vi "水样数据发送帧.vi"(10 "数据类别":u16(ring) items=["水样数据"=0, "标样数据"=1, "零点核查数据"=2, "跨度核查数据"=3, "环境变量"=4, "水样数据补传"=16, "标样核查数据补传"=17, "零点核查数据补传"=18, "跨度核查数据补传"=19], 11 "用户地址":string) -> (1 "非x？":bool, 2 "报文长度":i32, 3 "字符串":string)   [LabVIEW 2016, in "环境动力监测库.lvlib" / "NMEA.lvlib"]
uses:
  NMEA.lvlib
panel:
  out "data":T1 {"数组"."标识" items=["N"=1, "T"=2, "L"=3, "D"=4, "Z"=5, "M"=6, "hd"=7]; "数组"."污染物" items=["水温"=1, "浊度"=2, "DO"=3, "pH"=4, "ORP"=5, "比电导率"=6, "叶绿素a"=7, "氨氮"=8, "亚硝氮"=9, "硫化物"=10, "电压"=11, "温度"=12, "湿度"=13, "GPS经度"=14, "GPS纬度"=15, "BD经度"=16, "BD纬度"=17]; "数据类别" items=["水样数据"=0, "标样数据"=1, "零点核查数据"=2, "跨度核查数据"=3, "环境变量"=4, "水样数据补传"=16, "标样核查数据补传"=17, "零点核查数据补传"=18, "跨度核查数据补传"=19]}
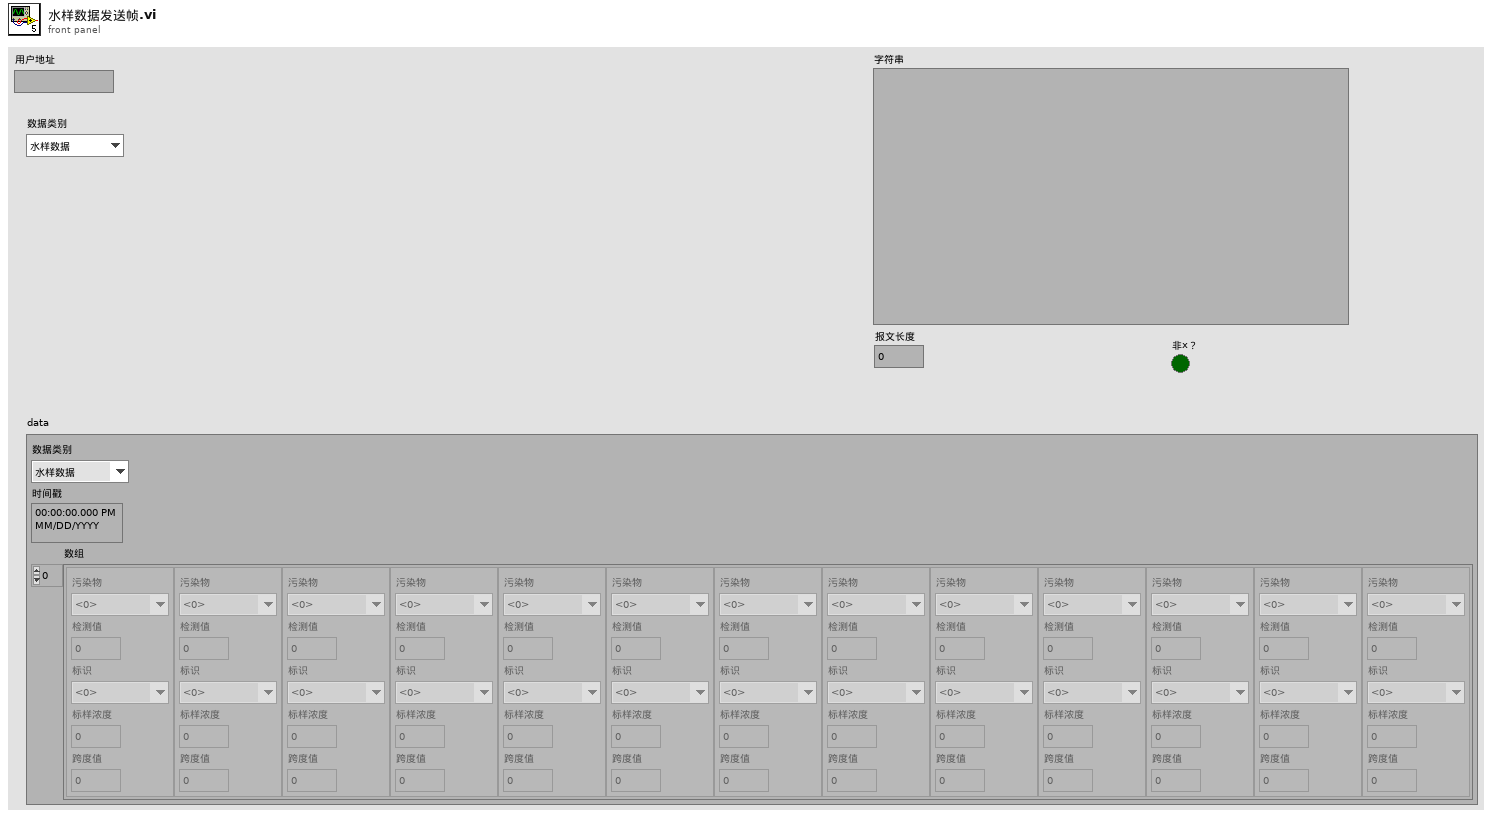
[diagram p1: front panel]
types:
  T1 = cluster{"数据类别":u16, "时间戳":timestamp, "数组":cluster{"污染物":u16, "检测值":dbl, "标识":u16, "标样浓度":dbl, "跨度值":dbl}[]}
  T2 = cluster{"污染物":u16, "检测值":dbl, "标识":u16, "标样浓度":dbl, "跨度值":dbl}[]
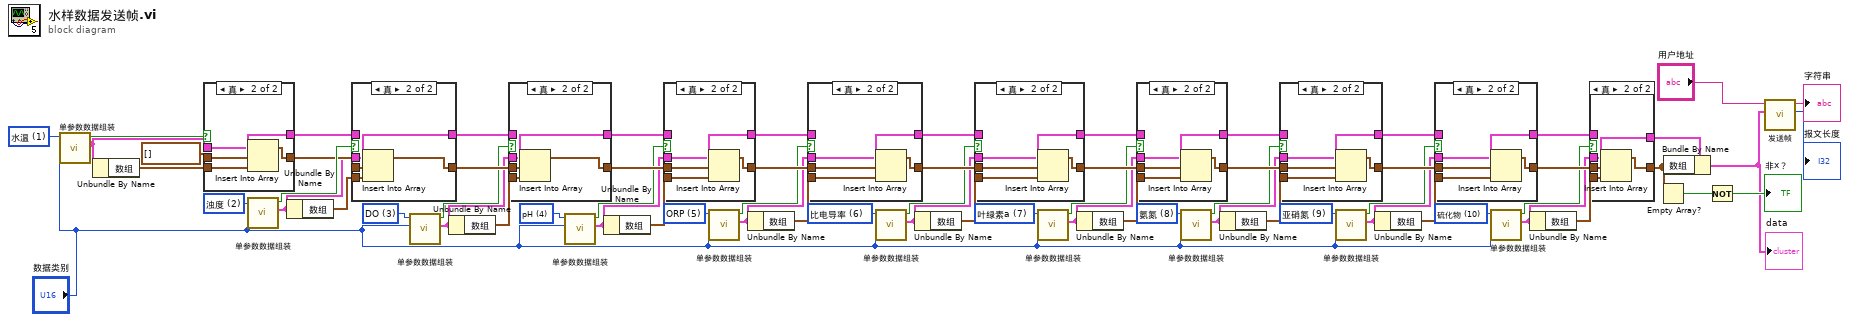
[diagram p0: block diagram]
diagram:
  w59 = u16 7 items=["水温"=1, "浊度"=2, "DO"=3, "pH"=4, "ORP"=5, "比电导率"=6, "叶绿素a"=7, "氨氮"=8, "亚硝氮"=9, "硫化物"=10, "经度"=11, "维度"=12, "电压"=13] ("污染物")
  w60 = u16 6 items=["水温"=1, "浊度"=2, "DO"=3, "pH"=4, "ORP"=5, "比电导率"=6, "叶绿素a"=7, "氨氮"=8, "亚硝氮"=9, "硫化物"=10, "经度"=11, "维度"=12, "电压"=13] ("污染物")
  w61 = u16 5 items=["水温"=1, "浊度"=2, "DO"=3, "pH"=4, "ORP"=5, "比电导率"=6, "叶绿素a"=7, "氨氮"=8, "亚硝氮"=9, "硫化物"=10, "经度"=11, "维度"=12, "电压"=13] ("污染物")
  w62 = u16 4 items=["水温"=1, "浊度"=2, "DO"=3, "pH"=4, "ORP"=5, "比电导率"=6, "叶绿素a"=7, "氨氮"=8, "亚硝氮"=9, "硫化物"=10, "经度"=11, "维度"=12, "电压"=13] ("污染物")
  w63 = u16 3 items=["水温"=1, "浊度"=2, "DO"=3, "pH"=4, "ORP"=5, "比电导率"=6, "叶绿素a"=7, "氨氮"=8, "亚硝氮"=9, "硫化物"=10, "经度"=11, "维度"=12, "电压"=13] ("污染物")
  w64 = u16 2 items=["水温"=1, "浊度"=2, "DO"=3, "pH"=4, "ORP"=5, "比电导率"=6, "叶绿素a"=7, "氨氮"=8, "亚硝氮"=9, "硫化物"=10, "经度"=11, "维度"=12, "电压"=13] ("污染物")
  w65 = u16 1 items=["水温"=1, "浊度"=2, "DO"=3, "pH"=4, "ORP"=5, "比电导率"=6, "叶绿素a"=7, "氨氮"=8, "亚硝氮"=9, "硫化物"=10, "经度"=11, "维度"=12, "电压"=13] ("污染物")
  w66 = u16 10 items=["水温"=1, "浊度"=2, "DO"=3, "pH"=4, "ORP"=5, "比电导率"=6, "叶绿素a"=7, "氨氮"=8, "亚硝氮"=9, "硫化物"=10, "经度"=11, "维度"=12, "电压"=13] ("污染物")
  w67 = u16 9 items=["水温"=1, "浊度"=2, "DO"=3, "pH"=4, "ORP"=5, "比电导率"=6, "叶绿素a"=7, "氨氮"=8, "亚硝氮"=9, "硫化物"=10, "经度"=11, "维度"=12, "电压"=13] ("污染物")
  w68 = u16 8 items=["水温"=1, "浊度"=2, "DO"=3, "pH"=4, "ORP"=5, "比电导率"=6, "叶绿素a"=7, "氨氮"=8, "亚硝氮"=9, "硫化物"=10, "经度"=11, "维度"=12, "电压"=13] ("污染物")
  n1 = call "单参数数据组装.vi"("数据类别"="数据类别", "污染物"=w65) -> ("data"=w28:T1, "布尔"=w58:bool)  [unwired: 8 in]
  n2 = Unbundle By Name(w28) -> ("数组"=w39:T2)
  n3 = case shown="真" w58 {
    tunnel: w39 -> [_ w74]
    tunnel: T2 [] ("数组") -> [w70 w73]
    tunnel: [w70 w72] -> w56
    tunnel: w28 -> [w69 w71]
    tunnel: [w69 w71] -> w27
    frame False {
    }
    frame True {
      n4 = Insert Into Array(array=w73, new element=w74) -> (w72:T2)  [unwired: 1 in]
    }
  }
  n5 = call "单参数数据组装.vi"("数据类别"="数据类别", "污染物"=w64) -> ("data"=w17:T1, "布尔"=w57:bool)  [unwired: 8 in]
  n6 = Unbundle By Name(w17) -> ("数组"=w38:T2)
  n7 = case shown="真" w57 {
    tunnel: w38 -> [_ w80]
    tunnel: w56 -> [w76 w79]
    tunnel: [w76 w78] -> w55
    tunnel: [w75 w77] -> w26
    tunnel: w27 -> [w75 _]
    tunnel: w17 -> [_ w77]
    frame False {
    }
    frame True {
      n8 = Insert Into Array(array=w79, new element=w80) -> (w78:T2)  [unwired: 1 in]
    }
  }
  n9 = call "单参数数据组装.vi"("数据类别"="数据类别", "污染物"=w63) -> ("data"=w16:T1, "布尔"=w50:bool)  [unwired: 8 in]
  n10 = Unbundle By Name(w16) -> ("数组"=w37:T2)
  n11 = case shown="真" w50 {
    tunnel: w37 -> [_ w86]
    tunnel: w55 -> [w82 w85]
    tunnel: [w82 w84] -> w54
    tunnel: w26 -> [w81 _]
    tunnel: [w81 w83] -> w25
    tunnel: w16 -> [_ w83]
    frame False {
    }
    frame True {
      n12 = Insert Into Array(array=w85, new element=w86) -> (w84:T2)  [unwired: 1 in]
    }
  }
  n13 = call "单参数数据组装.vi"("数据类别"="数据类别", "污染物"=w62) -> ("data"=w15:T1, "布尔"=w49:bool)  [unwired: 8 in]
  n14 = Unbundle By Name(w15) -> ("数组"=w36:T2)
  n15 = case shown="真" w49 {
    tunnel: w36 -> [_ w92]
    tunnel: w54 -> [w88 w91]
    tunnel: [w88 w90] -> w52
    tunnel: w25 -> [w87 _]
    tunnel: [w87 w89] -> w24
    tunnel: w15 -> [_ w89]
    frame False {
    }
    frame True {
      n16 = Insert Into Array(array=w91, new element=w92) -> (w90:T2)  [unwired: 1 in]
    }
  }
  n17 = call "单参数数据组装.vi"("数据类别"="数据类别", "污染物"=w61) -> ("data"=w14:T1, "布尔"=w48:bool)  [unwired: 8 in]
  n18 = Unbundle By Name(w14) -> ("数组"=w35:T2)
  n19 = case shown="真" w48 {
    tunnel: w35 -> [_ w98]
    tunnel: w52 -> [w94 w97]
    tunnel: [w94 w96] -> w53
    tunnel: w24 -> [w93 _]
    tunnel: [w93 w95] -> w23
    tunnel: w14 -> [_ w95]
    frame False {
    }
    frame True {
      n20 = Insert Into Array(array=w97, new element=w98) -> (w96:T2)  [unwired: 1 in]
    }
  }
  n21 = call "单参数数据组装.vi"("数据类别"="数据类别", "污染物"=w60) -> ("data"=w13:T1, "布尔"=w47:bool)  [unwired: 8 in]
  n22 = Unbundle By Name(w13) -> ("数组"=w34:T2)
  n23 = case shown="真" w47 {
    tunnel: w34 -> [_ w104]
    tunnel: w53 -> [w100 w103]
    tunnel: [w100 w102] -> w51
    tunnel: w23 -> [w99 _]
    tunnel: [w99 w101] -> w22
    tunnel: w13 -> [_ w101]
    frame False {
    }
    frame True {
      n24 = Insert Into Array(array=w103, new element=w104) -> (w102:T2)  [unwired: 1 in]
    }
  }
  n25 = call "单参数数据组装.vi"("数据类别"="数据类别", "污染物"=w59) -> ("data"=w12:T1, "布尔"=w46:bool)  [unwired: 8 in]
  n26 = Unbundle By Name(w12) -> ("数组"=w33:T2)
  n27 = case shown="真" w46 {
    tunnel: w33 -> [_ w110]
    tunnel: w51 -> [w106 w109]
    tunnel: [w106 w108] -> w43
    tunnel: w22 -> [w105 _]
    tunnel: [w105 w107] -> w21
    tunnel: w12 -> [_ w107]
    frame False {
    }
    frame True {
      n28 = Insert Into Array(array=w109, new element=w110) -> (w108:T2)  [unwired: 1 in]
    }
  }
  n29 = call "单参数数据组装.vi"("数据类别"="数据类别", "污染物"=w68) -> ("data"=w11:T1, "布尔"=w42:bool)  [unwired: 8 in]
  n30 = Unbundle By Name(w11) -> ("数组"=w32:T2)
  n31 = case shown="真" w42 {
    tunnel: w32 -> [_ w116]
    tunnel: w43 -> [w112 w115]
    tunnel: [w112 w114] -> w45
    tunnel: w21 -> [w111 _]
    tunnel: [w111 w113] -> w20
    tunnel: w11 -> [_ w113]
    frame False {
    }
    frame True {
      n32 = Insert Into Array(array=w115, new element=w116) -> (w114:T2)  [unwired: 1 in]
    }
  }
  n33 = call "单参数数据组装.vi"("数据类别"="数据类别", "污染物"=w67) -> ("data"=w10:T1, "布尔"=w41:bool)  [unwired: 8 in]
  n34 = Unbundle By Name(w10) -> ("数组"=w31:T2)
  n35 = case shown="真" w41 {
    tunnel: w31 -> [_ w122]
    tunnel: w45 -> [w118 w121]
    tunnel: [w118 w120] -> w44
    tunnel: w20 -> [w117 _]
    tunnel: [w117 w119] -> w19
    tunnel: w10 -> [_ w119]
    frame False {
    }
    frame True {
      n36 = Insert Into Array(array=w121, new element=w122) -> (w120:T2)  [unwired: 1 in]
    }
  }
  n37 = call "单参数数据组装.vi"("数据类别"="数据类别", "污染物"=w66) -> ("data"=w9:T1, "布尔"=w40:bool)  [unwired: 8 in]
  n38 = Unbundle By Name(w9) -> ("数组"=w30:T2)
  n39 = case shown="真" w40 {
    tunnel: w30 -> [_ w128]
    tunnel: w44 -> [w124 w127]
    tunnel: [w124 w126] -> w8
    tunnel: w19 -> [w123 _]
    tunnel: [w123 w125] -> w18
    tunnel: w9 -> [_ w125]
    frame False {
    }
    frame True {
      n40 = Insert Into Array(array=w127, new element=w128) -> (w126:T2)  [unwired: 1 in]
    }
  }
  n41 = Empty Array?(array=w8) -> (empty?=w4:bool)
  n42 = Bundle By Name(cluster=w18, "数组"=w8) -> (w1:T1)
  "data" <- w1
  n43 = Not(x=w4) -> (.not. x?=→"非x？":bool)
  n44 = call "发送帧.vi"("data"=w1, "用户地址"="用户地址") -> ("报文长度"=→"报文长度":i32, "字符串"=→"字符串":string)  [unwired: 8 in]
